vi "MenuBuild.vi"(4 "Button\n(Mouse Down?)":u16, 5 "Clipboard":refnum<vi>, 6 "withinSelection?":bool=TRUE, 7 "row type":T1, 8 "error in (no error)":errorcluster, 9 "Table CtlRef In":refnum<vi>, 10 "MenuRef In":refnum<k9>, 11 "LMenuCol in":refnum<class "ModeCol.lvclass">) -> (0 "error out":errorcluster, 1 "Table CtlRef Out":refnum<vi>, 2 "MenuRef Out":refnum<k9>, 3 "LMenuCol out":refnum<class "ModeCol.lvclass">)   [LabVIEW 2013, in "ModeCol.lvclass"]
doc: "Build menu items specific to Mode column. Presently this VI DOES MODIFY Column data."
uses:
  ModeCol.lvclass
  TypeDefs/RowType.ctl
  Column/Column.lvclass
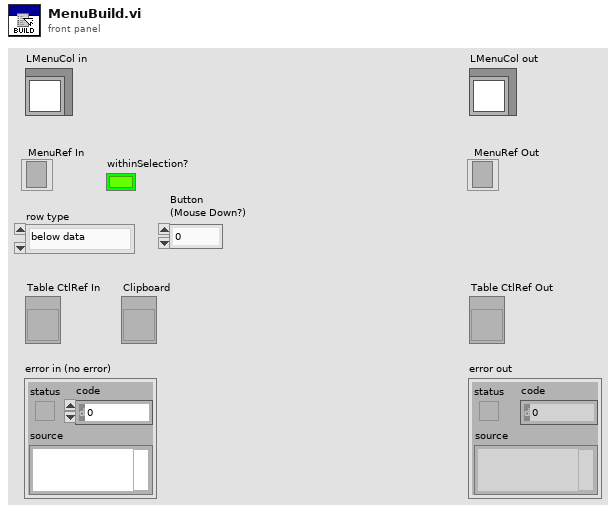
[diagram p1: front panel]
types:
  T1 = typedef "RowType.ctl" = enum16{"below data", "within data", "column header", "first row"}
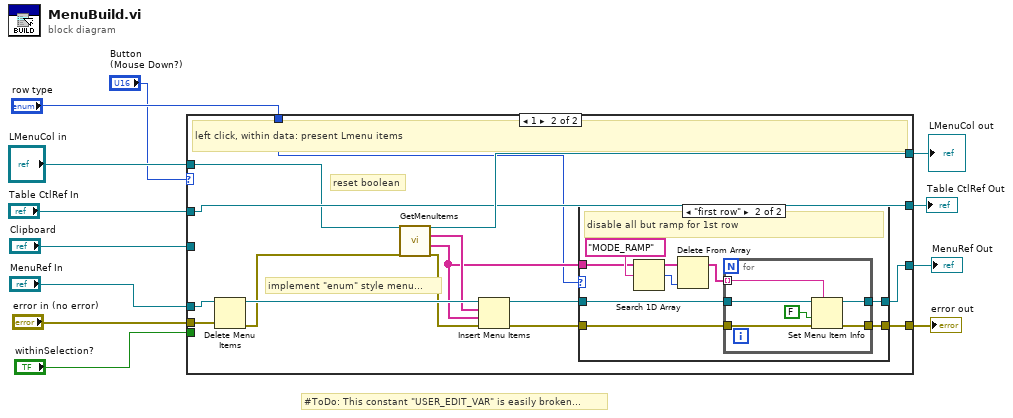
[diagram p0: block diagram]
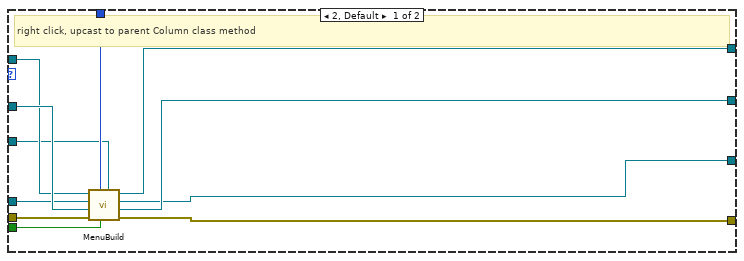
[diagram p2: hidden frame]
diagram:
  # "#ToDo: This constant \"USER_EDIT_VAR\" is easily broken..."
  n1 = case shown="1" "Button\n(Mouse Down?)" {
    tunnel: [w14 w30] -> w12
    tunnel: [w23 w32] -> w11
    tunnel: [w22 w35] -> w10
    tunnel: "row type" -> [w17 w26]
    tunnel: "Table CtlRef In" -> [w21 w32]
    tunnel: "MenuRef In" -> [w20 w38]
    tunnel: "LMenuCol in" -> [w19 w25]
    tunnel: "error in (no error)" -> [w18 w37]
    tunnel: [w15 w29] -> w7
    tunnel: "withinSelection?" -> [w16 _]
    tunnel: "Clipboard" -> [w13 _]
    frame 2, Default {
      # "right click, upcast to parent Column class method"
      n2 = call-parent "MenuBuild.vi"("Clipboard"=w13, "withinSelection?"=w16, "row type"=w17, "error in (no error)"=w18, "Table CtlRef In"=w21, "MenuRef In"=w20, "Column in"=w19) -> ("error out"=w14:errorcluster, "Table CtlRef Out"=w23:refnum<vi>, "MenuRef Out"=w15:refnum<k9>, "Column out"=w22:refnum<class "ModeCol.lvclass">)  [unwired: 1 in]
    }
    frame 1 {
      # "reset boolean"
      # "implement \"enum\" style menu..."
      # "left click, within data: present Lmenu items"
      n3 = Delete Menu Items(6:w37, 9:w38) -> (0:w24:errorcluster, 3:w36:refnum<k9>)  [unwired: 2 in]
      n4 = call "GetMenuItems.vi"("error in (no error)"=w24, "ModeCol in"=w25) -> ("error out"=w33:errorcluster, "LMenu tags"=w27:string[], "LMenu names"=w34:string[], "ModeCol out"=w35:refnum<class "ModeCol.lvclass">)  [unwired: 6 in]
      n5 = Insert Menu Items(6:w33, 7:w27, 8:w34, 9:w36) -> (0:w31:errorcluster, 3:w28:refnum<k9>)  [unwired: 2 in, 1 out]
      n6 = case shown="\"first row\"" w26 {
        tunnel: w31 -> [w39 w48]
        tunnel: [w39 w47] -> w30
        tunnel: [w40 w46] -> w29
        tunnel: w28 -> [w40 w45]
        tunnel: w27 -> [_ w42]
        frame Default {
          # "all modes allowed"
        }
        frame "first row" {
          # "disable all but ramp for 1st row"
          n7 = Search 1D Array(1D array=w42, element="MODE_RAMP") -> (index of element=w41:i32)  [unwired: 1 in]
          n8 = Delete From Array(array=w42, index=w41) -> (array with subset deleted=w44:string[])  [unwired: 1 in, 1 out]
          n9 = for {
            tunnel: w48 -> [w54]
            tunnel: [w53] -> w47
            tunnel: w44 -> [w49] mode=indexing
            tunnel: w45 -> [w51]
            tunnel: [w52] -> w46
            n10 = Set Menu Item Info(7:w49, 8:w54, 9:FALSE ("enabled"), 11:w51) -> (0:w53:errorcluster, 3:w52:refnum<k9>)  [unwired: 3 in]
          }
        }
      }
    }
  }
  "error out" <- w12
  "LMenuCol out" <- w10
  "MenuRef Out" <- w7
  "Table CtlRef Out" <- w11
